vi "Read Single Button Presses.vi"(0 "GEA2 Reference In":refnum<k24>, 11 "Error In":errorcluster) -> (4 "GEA2 Reference Out":refnum<k24>, 8 "Boolean array":bool[](array[boolean]), 15 "Error Out":errorcluster)   [LabVIEW 2016]
uses:
  C:/Automation/DLLs/PC Dot Net/GeaCommunication.dll
  Common/LabVIEW GEA2 Toolkit/LabVIEW_GEA2_Toolkit.lvlibp/type defs/ERD Read Data In.ctl
  Common/LabVIEW GEA2 Toolkit/LabVIEW_GEA2_Toolkit.lvlibp/type defs/Data Type.ctl
  Common/LabVIEW GEA2 Toolkit/LabVIEW_GEA2_Toolkit.lvlibp/type defs/Source_Destination.ctl
  Common/LabVIEW GEA2 Toolkit/LabVIEW_GEA2_Toolkit.lvlibp
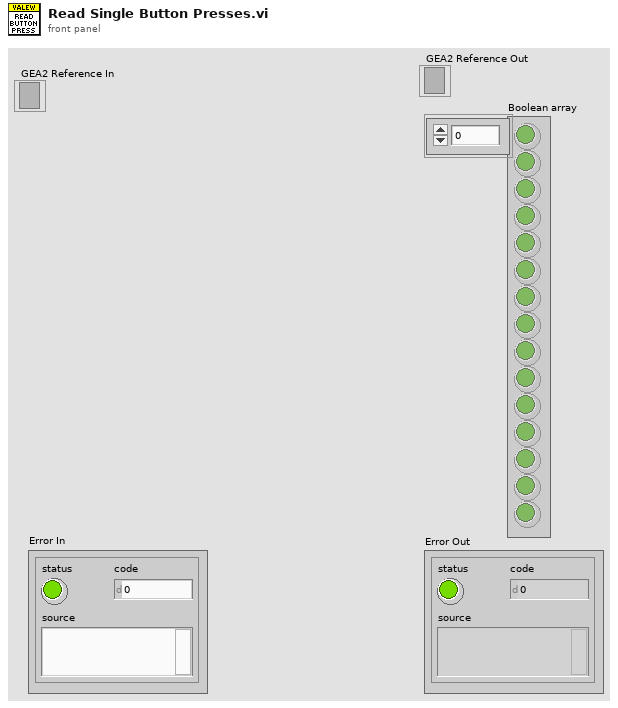
[diagram p1: front panel]
types:
  T1 = typedef "LabVIEW_GEA2_Toolkit.lvlibp/Source_Destination.ctl" = cluster{"Source":u8, "Destination":u8}
  T2 = typedef "LabVIEW_GEA2_Toolkit.lvlibp/ERD Read Data In.ctl" = cluster{"ERD Number":u16, "Data Type":T3}
  T3 = typedef "LabVIEW_GEA2_Toolkit.lvlibp/Data Type.ctl" = enum16{"string", "boolean", "uint8_t", "uint16_t", "uint32_t", "uint64_t", "int8_t", "int16_t", "int32_t", "int64_t"}
  T4 = typedef "LabVIEW_GEA2_Toolkit.lvlibp/ERD Read Data Out.ctl" = cluster{"ERD Number":u16, "Data":string}
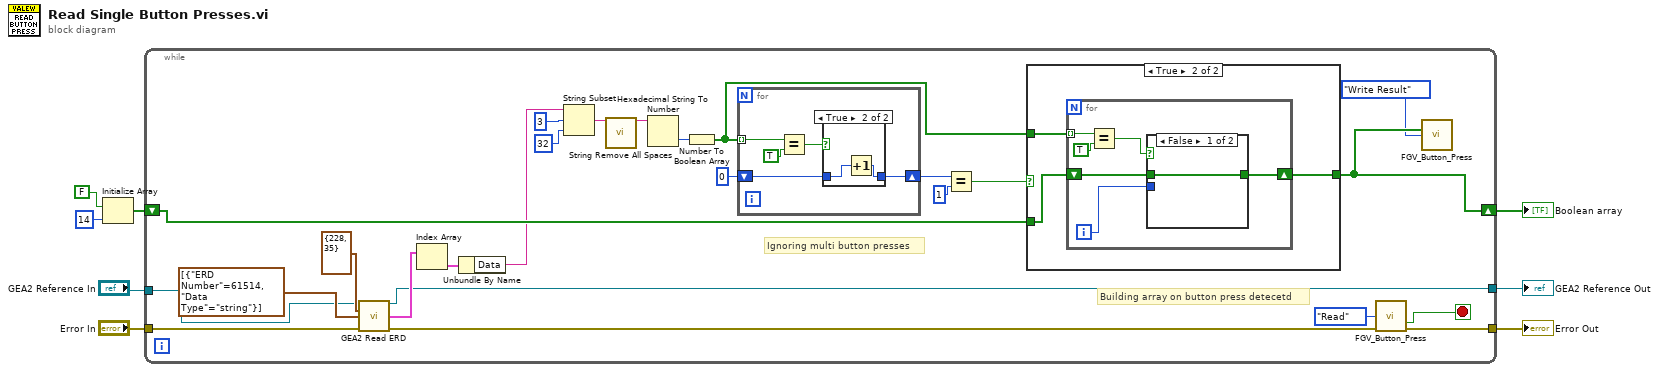
[diagram p0: block diagram]
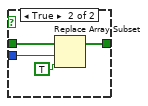
[diagram p3: hidden frame]
diagram:
  n1 = Initialize Array(FALSE, 14 ("dimension size")) -> (w6:bool[])
  n2 = while {
    shift-right: [w12] -> w2
    shift-left: w6 -> [w23]
    tunnel: "Error In" -> [w19]
    tunnel: [w21] -> w4
    tunnel: "GEA2 Reference In" -> [w16]
    tunnel: [w11] -> w3
    stop <- w22 stop-if-true
    # "Building array on button press detecetd"
    # "Ignoring multi button presses"
    n3 = call "GEA2 Read ERD.vi"("GEA2 Reference In"=w16, "GEA Inputs"=T1 {"Source"=228, "Destination"=35}, "Read ERD List"=T2[] [{"ERD Number"=61514, "Data Type"=enum."string"}], "Error In"=w19) -> ("GEA2 Reference Out"=w11:refnum<k24>, "ERD Data Out"=w15:T4[], "Error Out"=w18:errorcluster)  [unwired: 8 in, 1 out]
    n4 = Index Array(array=w15) -> (element=w14:T4)  [unwired: 1 in]
    n5 = Unbundle By Name(w14) -> ("Data"=w13:string)
    n6 = String Subset(string=w13, offset (0)=3, length (rest)=32 ("length (rest)")) -> (substring=w31:string)
    n7 = call "String Remove All Spaces.vi"("Input String"=w31) -> ("Spaces Removed"=w30:string)  [unwired: 13 in, 1 out]
    n8 = Hexadecimal String To Number(string=w30) -> (number=w29:u32)  [unwired: 2 in, 1 out]
    n9 = Number To Boolean Array(number=w29) -> (Boolean array=w24:bool[])
    n10 = for {
      tunnel: w24 -> [w49] mode=indexing
      shift-right: [w52] -> w27
      shift-left: 0 -> [w53]
      n11 = Equal?(x=w49, y=TRUE) -> (x = y?=w50:bool)
      n12 = case shown="True" w50 {
        tunnel: w53 -> [w54 w56]
        tunnel: [w54 w55] -> w52
        frame False {
        }
        frame True {
          n13 = Increment(x=w56) -> (x+1=w55:i32)
        }
      }
    }
    n14 = Equal?(x=w27, y=1) -> (x = y?=w25:bool)
    n15 = case shown="True" w25 {
      tunnel: w24 -> [_ w37]
      tunnel: [w34 w36] -> w12
      tunnel: w23 -> [w34 w35]
      frame False {
      }
      frame True {
        n16 = for {
          tunnel: w37 -> [w42] mode=indexing
          shift-right: [w40] -> w36
          shift-left: w35 -> [w39]
          i -> [w41]
          n17 = Equal?(x=w42, y=TRUE) -> (x = y?=w38:bool)
          n18 = case shown="False" w38 {
            tunnel: w41 -> [_ w48]
            tunnel: [w44 w46] -> w40
            tunnel: w39 -> [w44 w45]
            frame False {
            }
            frame True {
              n19 = Replace Array Subset(array=w45, new element=TRUE ("new element/subarray"), index=w48) -> (w46:bool[])
            }
          }
        }
      }
    }
    n20 = call "FGV_Button_Press.vi"("Action"=enum16{"Read", "Write Stop", "Write Result"}."Read", "Error In"=w18) -> ("Boolean Out"=w22:bool, "Error Out"=w21:errorcluster)  [unwired: 11 in, 1 out]
    n21 = call "FGV_Button_Press.vi"("Boolean array"=w12, "Action"=enum16{"Read", "Write Stop", "Write Result"}."Write Result") -> ()  [unwired: 11 in, 3 out]
  }
  "Boolean array" <- w2
  "Error Out" <- w4
  "GEA2 Reference Out" <- w3
